vi "Find Distance.vi"() -> ()   [LabVIEW 2015]
uses:
  <vilib>/vision/Measure.llb/Edge Options.ctl
  <vilib>/vision/Measure.llb/Edge Polarity.ctl
  <vilib>/vision/NI_Vision_Development_Module.lvlib
panel:
  out "Distance":sgl
  out "Image Out":T1(plugin-control)
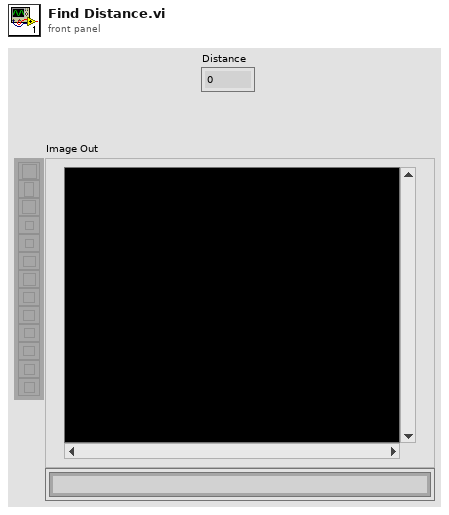
[diagram p1: front panel]
types:
  T1 = typedef "IMAQ Image.ctl" = refnum<image>
  T2 = typedef "Edge Options.ctl" = cluster{"Edge Polarity":T3, "Kernel Size":u32, "Width":u32, "Minimum Edge Strength":sgl, "Interpolation Type":enum32{"Zero Order", "Bilinear", "Quadratic", "Cubic", "Bilinear Fixed"}, "Data Processing Method":enum32{"Average", "Median"}}
  T3 = typedef "Edge Polarity.ctl" = u32
  T4 = cluster{"Search Direction":u32, "Edge Options":T2, "Show Search Area":bool, "Show Search Lines":bool, "Show Edges Found":bool, "Show Result":bool, "Search Area Color":u32, "Search Lines Color":u32, "Edge Locations Color":u32, "Result Color":u32, "Overlay Group Name":string}
  T5 = typedef "imagedata.ctl" = cluster{"image type":i32, "image depth":i32, "image":u8[], "mask":u8[], "colors":u32[], "Rectangle":cluster{"left":i16, "top":i16, "right":i16, "bottom":i16}}
  T6 = cluster{"left":i16, "top":i16, "right":i16, "bottom":i16}
  T7 = cluster{"left":i16, "top":i16, "right":i16, "bottom":i16, dbl}
  T8 = typedef "ROI Descriptor" = cluster{"Global Rectangle":i32[], "Contours":cluster{"ID":enum32{"External", "Internal"}, "Type":u32, "Coordinates":i32[]}[]}
  T9 = cluster{"Point1 (Pixels)":cluster{"X":sgl, "Y":sgl}, "Point2 (Pixels)":cluster{"X":sgl, "Y":sgl}, "Point1 (Real-World)":cluster{"X":sgl, "Y":sgl}, "Point2 (Real-World)":cluster{"X":sgl, "Y":sgl}, "Angle (Pixel)":dbl, "Angle (Real-World)":dbl, "Score":dbl, "Straightness":dbl, "Average SNR (db)":dbl, "Calibration Valid":bool}[]
  T10 = cluster{"Straight Edges[0]":cluster{"Point1 (Pixels)":cluster{"X":sgl, "Y":sgl}, "Point2 (Pixels)":cluster{"X":sgl, "Y":sgl}, "Point1 (Real-World)":cluster{"X":sgl, "Y":sgl}, "Point2 (Real-World)":cluster{"X":sgl, "Y":sgl}, "Angle (Pixel)":dbl, "Angle (Real-World)":dbl, "Score":dbl, "Straightness":dbl, "Average SNR (db)":dbl, "Calibration Valid":bool}, "Straight Edges[1]":cluster{"Point1 (Pixels)":cluster{"X":sgl, "Y":sgl}, "Point2 (Pixels)":cluster{"X":sgl, "Y":sgl}, "Point1 (Real-World)":cluster{"X":sgl, "Y":sgl}, "Point2 (Real-World)":cluster{"X":sgl, "Y":sgl}, "Angle (Pixel)":dbl, "Angle (Real-World)":dbl, "Score":dbl, "Straightness":dbl, "Average SNR (db)":dbl, "Calibration Valid":bool}, "Straight Edges[2]":cluster{"Point1 (Pixels)":cluster{"X":sgl, "Y":sgl}, "Point2 (Pixels)":cluster{"X":sgl, "Y":sgl}, "Point1 (Real-World)":cluster{"X":sgl, "Y":sgl}, "Point2 (Real-World)":cluster{"X":sgl, "Y":sgl}, "Angle (Pixel)":dbl, "Angle (Real-World)":dbl, "Score":dbl, "Straightness":dbl, "Average SNR (db)":dbl, "Calibration Valid":bool}, "Straight Edges[3]":cluster{"Point1 (Pixels)":cluster{"X":sgl, "Y":sgl}, "Point2 (Pixels)":cluster{"X":sgl, "Y":sgl}, "Point1 (Real-World)":cluster{"X":sgl, "Y":sgl}, "Point2 (Real-World)":cluster{"X":sgl, "Y":sgl}, "Angle (Pixel)":dbl, "Angle (Real-World)":dbl, "Score":dbl, "Straightness":dbl, "Average SNR (db)":dbl, "Calibration Valid":bool}, "Straight Edges[4]":cluster{"Point1 (Pixels)":cluster{"X":sgl, "Y":sgl}, "Point2 (Pixels)":cluster{"X":sgl, "Y":sgl}, "Point1 (Real-World)":cluster{"X":sgl, "Y":sgl}, "Point2 (Real-World)":cluster{"X":sgl, "Y":sgl}, "Angle (Pixel)":dbl, "Angle (Real-World)":dbl, "Score":dbl, "Straightness":dbl, "Average SNR (db)":dbl, "Calibration Valid":bool}, "Straight Edges[5]":cluster{"Point1 (Pixels)":cluster{"X":sgl, "Y":sgl}, "Point2 (Pixels)":cluster{"X":sgl, "Y":sgl}, "Point1 (Real-World)":cluster{"X":sgl, "Y":sgl}, "Point2 (Real-World)":cluster{"X":sgl, "Y":sgl}, "Angle (Pixel)":dbl, "Angle (Real-World)":dbl, "Score":dbl, "Straightness":dbl, "Average SNR (db)":dbl, "Calibration Valid":bool}, "Straight Edges[6]":cluster{"Point1 (Pixels)":cluster{"X":sgl, "Y":sgl}, "Point2 (Pixels)":cluster{"X":sgl, "Y":sgl}, "Point1 (Real-World)":cluster{"X":sgl, "Y":sgl}, "Point2 (Real-World)":cluster{"X":sgl, "Y":sgl}, "Angle (Pixel)":dbl, "Angle (Real-World)":dbl, "Score":dbl, "Straightness":dbl, "Average SNR (db)":dbl, "Calibration Valid":bool}, "Straight Edges[7]":cluster{"Point1 (Pixels)":cluster{"X":sgl, "Y":sgl}, "Point2 (Pixels)":cluster{"X":sgl, "Y":sgl}, "Point1 (Real-World)":cluster{"X":sgl, "Y":sgl}, "Point2 (Real-World)":cluster{"X":sgl, "Y":sgl}, "Angle (Pixel)":dbl, "Angle (Real-World)":dbl, "Score":dbl, "Straightness":dbl, "Average SNR (db)":dbl, "Calibration Valid":bool}, "Straight Edges[8]":cluster{"Point1 (Pixels)":cluster{"X":sgl, "Y":sgl}, "Point2 (Pixels)":cluster{"X":sgl, "Y":sgl}, "Point1 (Real-World)":cluster{"X":sgl, "Y":sgl}, "Point2 (Real-World)":cluster{"X":sgl, "Y":sgl}, "Angle (Pixel)":dbl, "Angle (Real-World)":dbl, "Score":dbl, "Straightness":dbl, "Average SNR (db)":dbl, "Calibration Valid":bool}}
  T11 = cluster{"X":sgl, "Y":sgl, "right":i16, "bottom":i16, dbl}
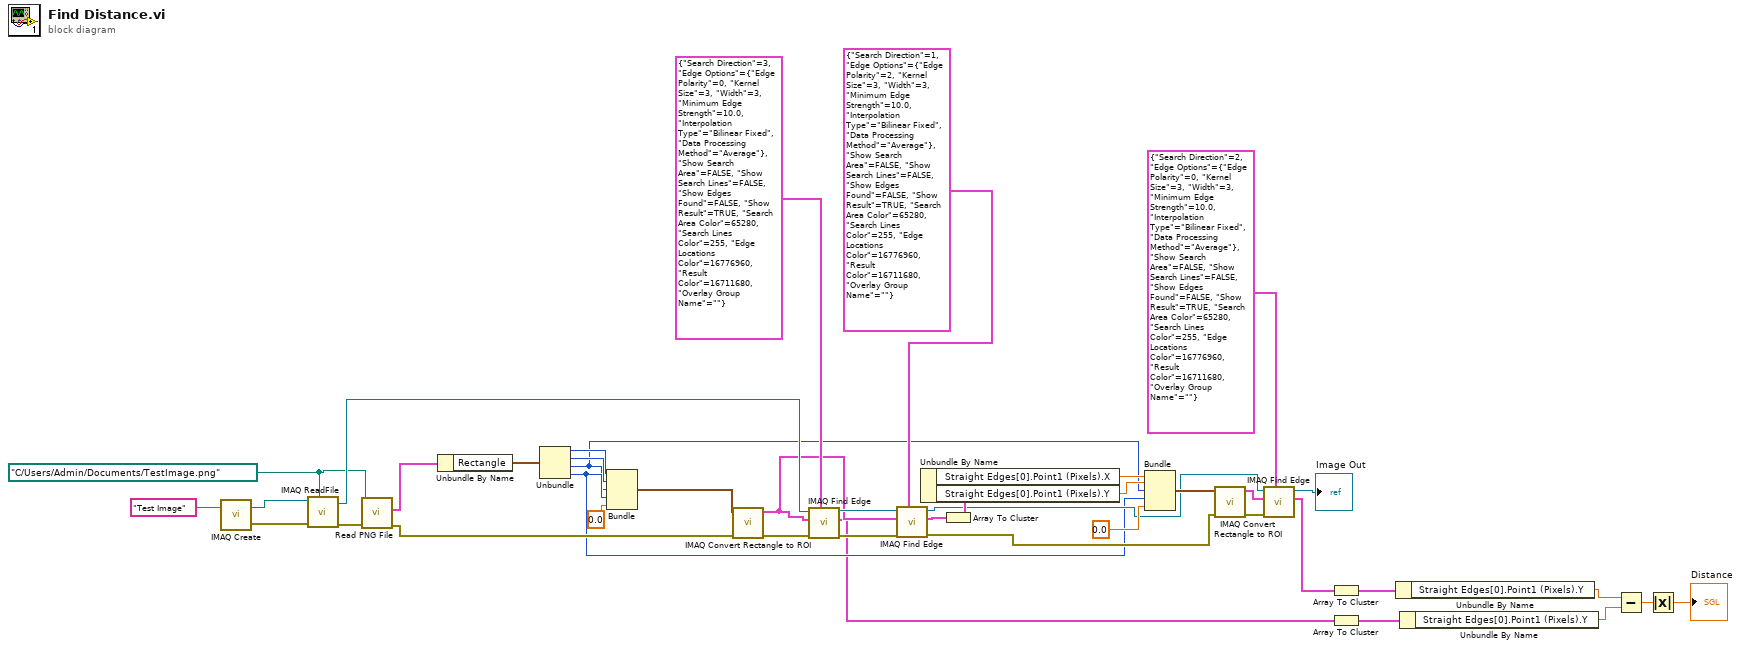
[diagram p0: block diagram]
diagram:
  w36 = path "C:/Users/Admin/Documents/TestImage.png" ("File Path")
  n1 = call "IMAQ Create"("Image Name"="Test Image") -> ("New Image"=w40:T1, "error out"=w39:errorcluster)  [unwired: 4 in]
  n2 = call "IMAQ ReadFile"("File Path"=w36, "error in (no error)"=w39, "Image"=w40) -> ("error out"=w35:errorcluster, "Image Out"=w37:T1)  [unwired: 4 in, 3 out]
  n3 = call <vilib>:"Read PNG File.vi"("error in (no error)"=w35, "path to PNG file"=w36) -> ("error out"=w30:errorcluster, "image data"=w34:T5)  [unwired: 7 in, 1 out]
  n4 = Unbundle By Name(w34) -> ("Rectangle"=w33:T6)
  n5 = Unbundle(w33) -> ("left"=w21:i16, "top"=w22:i16, "right"=w9:i16, "bottom"=w10:i16)
  n6 = Bundle("left"=w21, "top"=w22, "right"=w9, "bottom"=w10, 0.0) -> (w31:T7)  [unwired: 1 in]
  n7 = call "IMAQ Convert Rectangle to ROI"("error in (no error)"=w30, "Rectangle"=w31) -> ("error out"=w29:errorcluster, "ROI Descriptor"=w26:T8)  [unwired: 7 in]
  n8 = call "IMAQ Find Edge"("Options"=T4 {"Search Direction"=3, "Edge Options"={"Edge Polarity"=0, "Kernel Size"=3, "Width"=3, "Minimum Edge Strength"=10.0, "Interpolation Type"=enum."Bilinear Fixed", "Data Processing Method"=enum."Average"}, "Show Search Area"=FALSE, "Show Search Lines"=FALSE, "Show Edges Found"=FALSE, "Show Result"=TRUE, "Search Area Color"=65280, "Search Lines Color"=255, "Edge Locations Color"=16776960, "Result Color"=16711680, "Overlay Group Name"=""}, "error in (no error)"=w29, "ROI Descriptor"=w26, "Image"=w37) -> ("error out"=w27:errorcluster, "Straight Edges"=w8:T9, "Image Out"=w28:T1)  [unwired: 4 in, 1 out]
  n9 = call "IMAQ Find Edge"("Options"=T4 {"Search Direction"=1, "Edge Options"={"Edge Polarity"=2, "Kernel Size"=3, "Width"=3, "Minimum Edge Strength"=10.0, "Interpolation Type"=enum."Bilinear Fixed", "Data Processing Method"=enum."Average"}, "Show Search Area"=FALSE, "Show Search Lines"=FALSE, "Show Edges Found"=FALSE, "Show Result"=TRUE, "Search Area Color"=65280, "Search Lines Color"=255, "Edge Locations Color"=16776960, "Result Color"=16711680, "Overlay Group Name"=""}, "error in (no error)"=w27, "ROI Descriptor"=w26, "Image"=w28) -> ("error out"=w18:errorcluster, "Straight Edges"=w24:T9, "Image Out"=w15:T1)  [unwired: 4 in, 1 out]
  n10 = Array To Cluster(array=w24) -> (cluster=w23:T10)
  n11 = Unbundle By Name(w23) -> ("Straight Edges[0].Point1 (Pixels).X"=w12:sgl, "Straight Edges[0].Point1 (Pixels).Y"=w11:sgl)
  n12 = Bundle("X"=w12, "Y"=w11, "right"=w9, "bottom"=w10, 0.0) -> (w19:T11)  [unwired: 1 in]
  n13 = call "IMAQ Convert Rectangle to ROI"("error in (no error)"=w18, "Rectangle"=w19) -> ("error out"=w17:errorcluster, "ROI Descriptor"=w16:T8)  [unwired: 7 in]
  n14 = call "IMAQ Find Edge"("Options"=T4 {"Search Direction"=2, "Edge Options"={"Edge Polarity"=0, "Kernel Size"=3, "Width"=3, "Minimum Edge Strength"=10.0, "Interpolation Type"=enum."Bilinear Fixed", "Data Processing Method"=enum."Average"}, "Show Search Area"=FALSE, "Show Search Lines"=FALSE, "Show Edges Found"=FALSE, "Show Result"=TRUE, "Search Area Color"=65280, "Search Lines Color"=255, "Edge Locations Color"=16776960, "Result Color"=16711680, "Overlay Group Name"=""}, "error in (no error)"=w17, "ROI Descriptor"=w16, "Image"=w15) -> ("Straight Edges"=w6:T9, "Image Out"=→"Image Out":T1)  [unwired: 4 in, 2 out]
  n15 = Array To Cluster(array=w6) -> (cluster=w5:T10)
  n16 = Array To Cluster(array=w8) -> (cluster=w7:T10)
  n17 = Unbundle By Name(w5) -> ("Straight Edges[0].Point1 (Pixels).Y"=w3:sgl)
  n18 = Unbundle By Name(w7) -> ("Straight Edges[0].Point1 (Pixels).Y"=w4:sgl)
  n19 = Subtract(x=w3, y=w4) -> (x-y=w2:sgl)
  n20 = Absolute Value(x=w2) -> (abs(x)=→"Distance":sgl)
